vi "Subtopics to XML.vi"(1 "Topic in":refnum<class "Topic.lvclass">) -> (0 "tagged string":string)   [LabVIEW 2020, in "Topic.lvclass"]
uses:
  Topic.lvclass
  Topic.lvclass/Topic.ctl
  XMLInterface/XmlInterface.lvclass
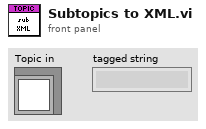
[diagram p1: front panel]
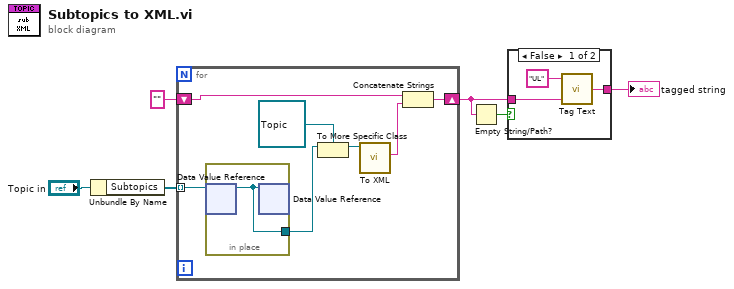
[diagram p0: block diagram]
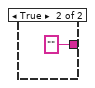
[diagram p2: hidden frame]
diagram:
  n1 = Unbundle By Name("Topic in") -> ("Subtopics"=w3:refnum<data-value>[])
  n2 = for {
    tunnel: w3 -> [w13] mode=indexing
    shift-right: [w12] -> w2
    shift-left: "" -> [w11]
    n3 = in-place {
      in-place-border: [w14] -> w10
      n4 = in-place-dvr #1(w13) -> (w14:refnum<class>)  [unwired: 1 out]
      n5 = in-place-dvr #1(w14) -> ()  [unwired: 2 out]
    }
    n6 = To More Specific Class(target class=refnum<class "Topic.lvclass"> refnum ("Topic.lvclass"), reference=w10) -> (specific class reference=w8:refnum<class "Topic.lvclass">)  [unwired: 1 in, 1 out]
    n7 = call-dynamic "To XML.vi"("Topic in"=w8) -> ("XML String"=w7:string)  [unwired: 8 in, 2 out]
    n8 = Concatenate Strings(w11, w7) -> (w12:string)
  }
  n9 = Empty String/Path?(string/path=w2) -> (empty?=w1:bool)
  n10 = case shown="False" w1 {
    tunnel: [w17 "" ("tagged string")] -> w5
    tunnel: w2 -> [w15 _]
    frame False {
      n11 = call "Tag Text.vi"("Value"=w15, "Tag"="UL") -> ("tagged string"=w17:string)  [unwired: 3 in]
    }
    frame True {
    }
  }
  "tagged string" <- w5
